vi "Byte Buffer.Set Buffer.vi"(8 "error in (no error)":errorcluster, 10 "buffer":string, 11 "Byte Buffer in":refnum<class "Byte Buffer.lvclass">) -> (0 "error out":errorcluster, 3 "Byte Buffer out":refnum<class "Byte Buffer.lvclass">)   [LabVIEW 2016, in "VeriStand Data.lvlib" / "Byte Buffer.lvclass"]
doc: "Gets the raw string buffer from the provided Byte Buffer class."
uses:
  Byte Buffer.lvclass
  Byte Buffer.lvclass/Byte Buffer.ctl
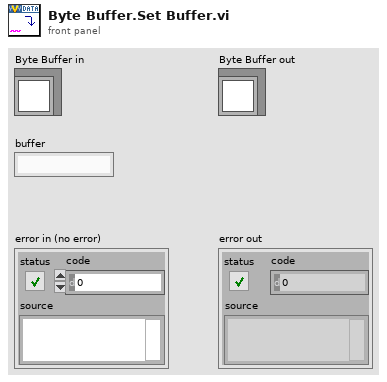
[diagram p1: front panel]
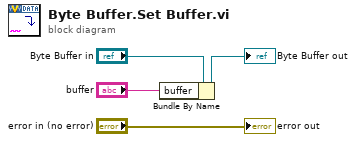
[diagram p0: block diagram]
diagram:
  n1 = Bundle By Name(cluster="Byte Buffer in", "buffer"="buffer") -> (→"Byte Buffer out":refnum<class "Byte Buffer.lvclass">)
  "error out" <- "error in (no error)"
